vi "TestAnalogFrontEnd.vi"(8 "error in":errorcluster, 11 "nWhichChan":i32=1) -> (0 "error out":errorcluster, 3 "Return Code":i32)   [LabVIEW 2015]
doc: "This test will check the front end to confirm is was manufactured correctly. It forces the hardware to the 10 V scale, and requires a square wave input (2.5 V, 62.5 Hertz).\n\nint nWhichChan – integer value with which channel to test (values 1 –4).\n\nThis function returns a 0 if the function completed successfully. A non-zero return code will indicate error."
uses:
  ScannerDiagDLL.dll
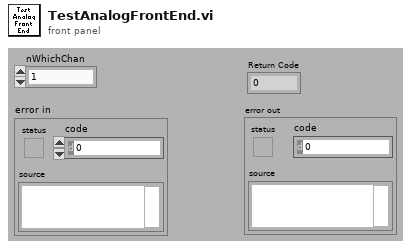
[diagram p1: front panel]
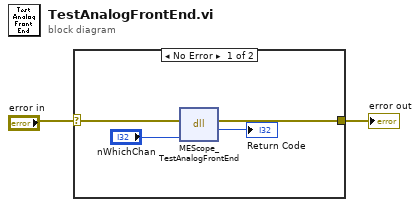
[diagram p0: block diagram]
diagram:
  n1 = case shown="No Error" "error in" {
    selector: "error in" -> [w5 w7]
    tunnel: [w4 w7] -> w1
    frame No Error {
      n2 = dll-call lib="C:/SNAPON/ModisEdge/TabletScope/Test Sequence/Code Modules/DLL/ScannerDiagDLL.dll" fn="MEScope_TestAnalogFrontEnd"(error in=w5, "nWhichChan"="nWhichChan") -> (error out=w4:errorcluster, "return type"=→"Return Code":i32)  [unwired: 3 in, 1 out]
    }
    frame Error {
    }
  }
  "error out" <- w1
